vi "Scaledata(Array).vi"(5 "Offset":dbl, 7 "Factor":dbl, 11 "Data in":dbl[](array[numeric])) -> (3 "Data out":dbl[](array[numeric]))   [LabVIEW 2014]
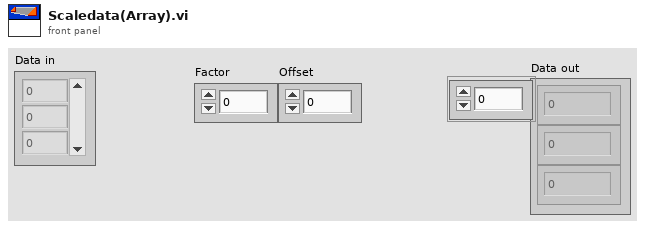
[diagram p1: front panel]
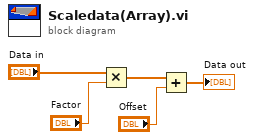
[diagram p0: block diagram]
diagram:
  n1 = Multiply(x="Data in", y="Factor") -> (x*y=w4:dbl[])
  n2 = Add(x=w4, y="Offset") -> (x+y=→"Data out":dbl[])
